vi "Enable Variable Forcing.vi"(6 "error in (no error)":errorcluster, 9 "target address (localhost)":string="localhost") -> (0 "error out":errorcluster)   [LabVIEW 2020]
doc: "Enables forcing for I/O variables and I/O aliases on the target."
uses:
  <resource>/objmgr/ni.var.rc
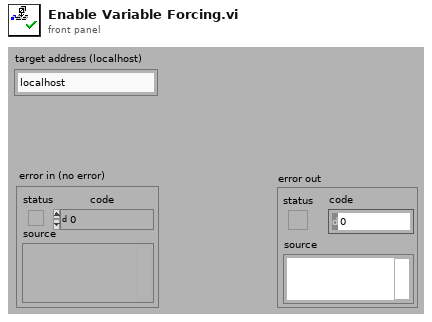
[diagram p1: front panel]
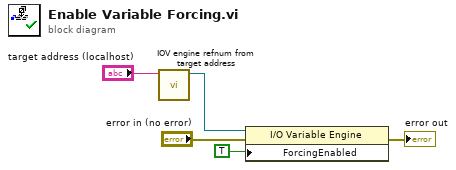
[diagram p0: block diagram]
diagram:
  n1 = call <vilib>:"IOV engine refnum from target address.vi"("target address"="target address (localhost)") -> ("reference out"=w5:refnum<k21>)  [unwired: 10 in]
  n2 = property class="I/O Variable Engine"(reference=w5, error in="error in (no error)", "ForcingEnabled"=TRUE ("IO Forcing Enabled")) -> (error out=→"error out":errorcluster)  [unwired: 1 out]
